vi "Test SigMan Control.vi"() -> ()   [LabVIEW 2020]
uses:
  Controls/SignalManager/SignalManager.xctl
  Classes/SignalManager/SignalManager.lvclass
  Controls/SignalManager/PeriodDisplay.ctl
  Classes/SignalManager/SignalManager.lvclass/SignalManager.ctl
  Classes/SignalManager/Read Error.vi
panel:
  in  "Frame (ms)":dbl
  out "Elapsed time (ms)":u32
  out "Graph":dbl[][](graph)
  out "Error":string
  in  "Read":bool
  in  "Write":bool
  in  "stop":bool
  in  "SigMan":refnum<class "SignalManager.lvclass">(xcontrol)
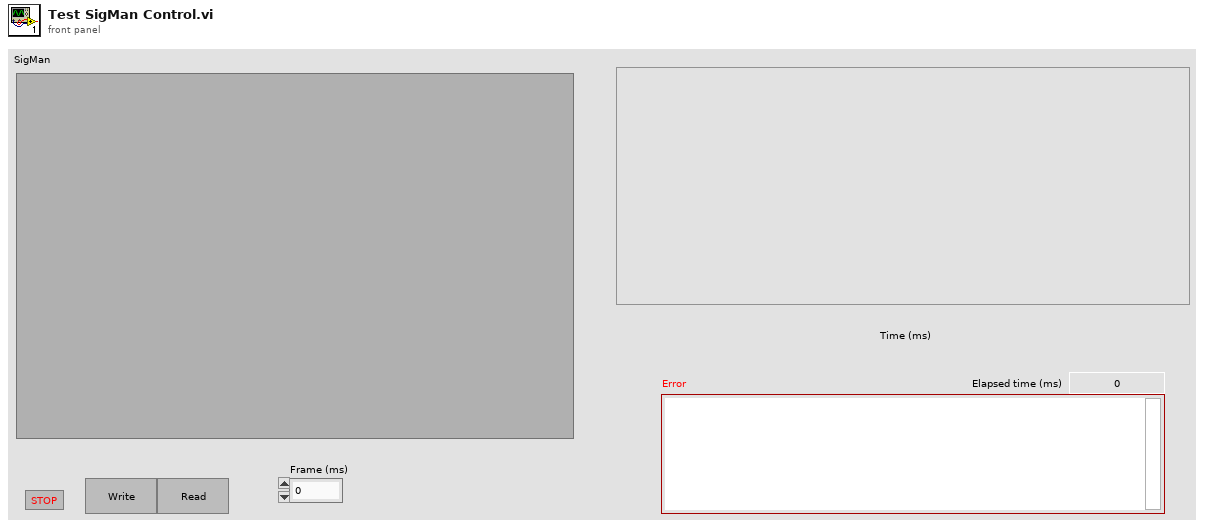
[diagram p1: front panel]
types:
  T1 = typedef "SignalManager.xctl/PeriodDisplay.ctl" = enum16{"Interval", "RepRate", "Both"}
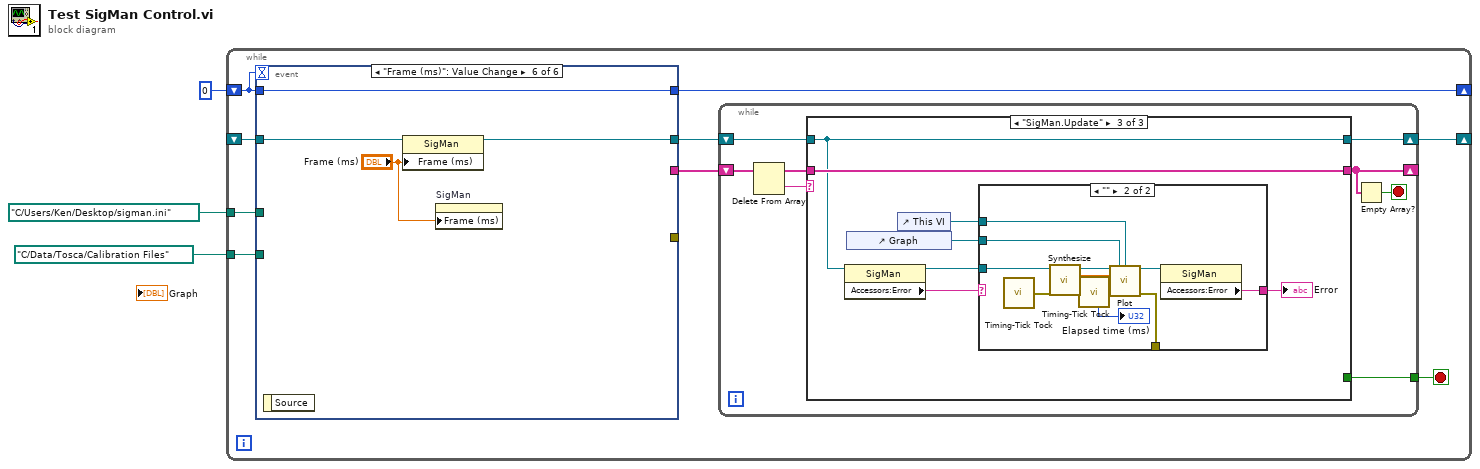
[diagram p0: block diagram]
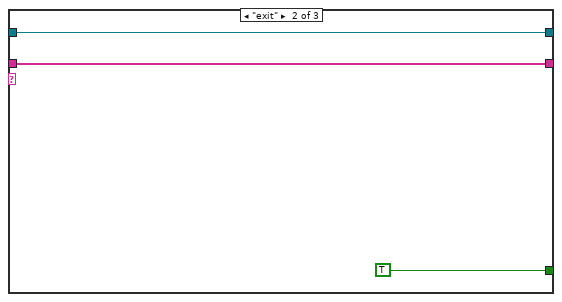
[diagram p3: hidden frame]
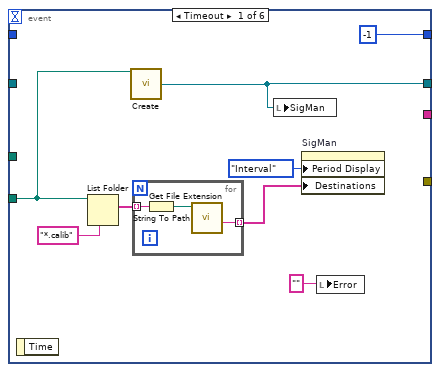
[diagram p5: hidden frame]
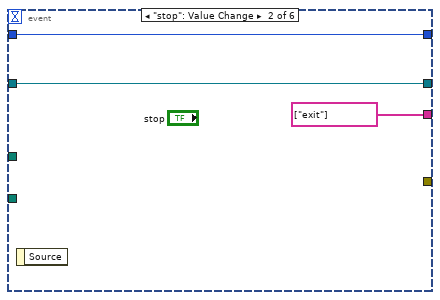
[diagram p6: hidden frame]
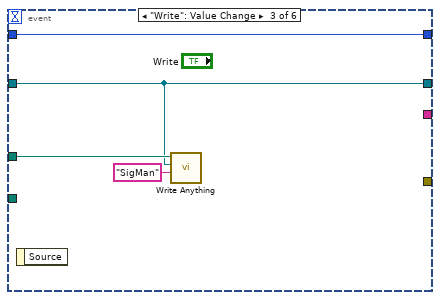
[diagram p7: hidden frame]
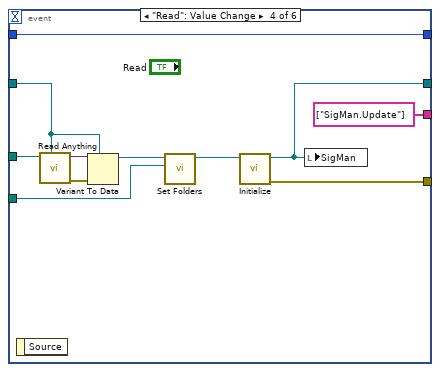
[diagram p8: hidden frame]
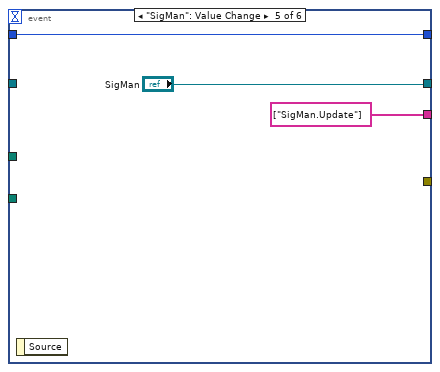
[diagram p9: hidden frame]
diagram:
  n1 = while {
    shift-right: [w11] -> _
    shift-left: 0 -> [w12]
    tunnel: path "C:/Users/Ken/Desktop/sigman.ini" ("Path (dialog)") -> [w10]
    shift-right: [w7] -> _
    shift-left: _ -> [w6]
    tunnel: path "C:/Data/Tosca/Calibration Files" ("Path (dialog)") -> [w4]
    stop <- w5 stop-if-true
    n2 = event shown="[5] \"Frame (ms)\": Value Change" {
      selector: _ -> [_ _ _ _ _ _]
      dyn-events: _ -> [_ _ _ _ _ _]
      timeout: w12 -> [_ _ _ _ _ _]
      tunnel: w12 -> [_ w59 w63 w74 w77 w81]
      tunnel: [-1 w59 w63 w74 w77 w81] -> w11
      tunnel: w10 -> [_ _ w62 w73 _ _]
      tunnel: [w51 w57 w61 w68 "SigMan" w79] -> w8
      tunnel: [_ string[] ["exit"] _ string[] ["SigMan.Update"] string[] ["SigMan.Update"] _] -> w9
      tunnel: w6 -> [_ w57 w61 w70 _ w80]
      tunnel: w4 -> [w50 _ _ w64 _ _]
      tunnel: [_ _ _ w67 _ _] -> _
      event Timeout {
        n3 = event-data() -> ()  [unwired: 1 in, 1 out]
        n4 = List Folder(path=w50, pattern="*.calib") -> (filenames=w48:string[])  [unwired: 2 in, 3 out]
        n5 = call "Create.vi"("Cal Folder"=w50) -> ("SigMan"=w51:refnum<class "SignalManager.lvclass">)  [unwired: 14 in]
        n6 = for {
          tunnel: w48 -> [w55] mode=indexing
          tunnel: [w56] -> w47 mode=indexing
          n7 = String To Path(string=w55) -> (path=w54:path)
          n8 = call <vilib>:"Get File Extension.vi"("file"=w54) -> ("filename without extension"=w56:string)  [unwired: 6 in, 4 out]
        }
        n9 = local write "SigMan"(w51) -> ()
        n10 = property on="SigMan" class="SignalManager (strict)"("Period Display"=PeriodDisplay."Interval", "Destinations"=w47) -> ()  [unwired: 2 in, 2 out]
        n11 = local write "Error"("" ("Error")) -> ()
      }
      event "stop": Value Change {
        n12 = event-data() -> ()  [unwired: 1 in, 1 out]
      }
      event "Write": Value Change {
        n13 = event-data() -> ()  [unwired: 1 in, 1 out]
        n14 = call "Write Anything.vi"("Section Name (Name of \"Anything\")"="SigMan" ("Section Name (Name of \"Anything\")"), "Anything"=w61, "Path (dialog)"=w62) -> ()  [unwired: 7 in, 2 out]
      }
      event "Read": Value Change {
        n15 = event-data() -> ()  [unwired: 1 in, 1 out]
        n16 = call "Read Anything.vi"("Type of Anything"=w70, "Path (dialog)"=w73) -> ("Error Out"=w72:errorcluster, "Anything"=w71:variant)  [unwired: 7 in, 1 out]
        n17 = Variant To Data(error in=w72, type=w70, Variant=w71) -> (data=w66:refnum<class "SignalManager.lvclass">)  [unwired: 1 out]
        n18 = call "Set Folders.vi"("Calibration folder"=w64, "SigMan in"=w66) -> ("SigMan out"=w65:refnum<class "SignalManager.lvclass">)  [unwired: 8 in, 1 out]
        n19 = call "Initialize.vi"("SigMan in"=w65) -> ("error out"=w67:errorcluster, "SigMan out"=w68:refnum<class "SignalManager.lvclass">)  [unwired: 9 in]
        n20 = local write "SigMan"(w68) -> ()
      }
      event "SigMan": Value Change {
        n21 = event-data() -> ()  [unwired: 1 in, 1 out]
      }
      event "Frame (ms)": Value Change {
        n22 = event-data() -> ()  [unwired: 1 in, 1 out]
        n23 = property class="SigMan"(reference=w80, "Frame (ms)"="Frame (ms)") -> (reference out=w79:refnum<class "SignalManager.lvclass">)  [unwired: 1 in, 1 out]
        n24 = property on="SigMan" class="SignalManager (strict)"("Frame (ms)"="Frame (ms)") -> ()  [unwired: 2 in, 2 out]
      }
    }
    n25 = while {
      shift-right: [w17] -> _
      shift-left: w9 -> [w20]
      shift-right: [w14] -> w7
      shift-left: w8 -> [w15]
      tunnel: [w13] -> w5
      stop <- w16 stop-if-true
      n26 = Delete From Array(array=w20) -> (deleted portion=w18:string, array with subset deleted=w19:string[])  [unwired: 2 in]
      n27 = case shown="\"SigMan.Update\"" w18 {
        tunnel: w19 -> [w22 w25 w32]
        tunnel: [w22 w25 w32] -> w17
        tunnel: w15 -> [w21 w24 w31]
        tunnel: [w21 w24 w31] -> w14
        tunnel: [_ TRUE _] -> w13
        frame "", Default {
        }
        frame "exit" {
        }
        frame "SigMan.Update" {
          n28 = property class="SigMan"(reference=w31) -> (reference out=w29:refnum<class "SignalManager.lvclass">, "Accessors:Error"=w30:string)  [unwired: 1 in, 1 out]
          n29 = control-ref of="Graph"() -> (w28:refnum<vi>)
          n30 = control-ref of="This VI"() -> (w27:refnum<vi>)
          n31 = case shown="\"\"" w30 {
            selector: w30 -> [w33 _]
            tunnel: w29 -> [_ w45]
            tunnel: w28 -> [_ w42]
            tunnel: w27 -> [_ w41]
            tunnel: [w33 w38] -> w26
            tunnel: [_ w37] -> _
            frame "error", Default {
            }
            frame "" {
              n32 = call "Timing-Tick Tock.vi"() -> ("error out"=w36:errorcluster)  [unwired: 6 in, 1 out]
              n33 = call "Synthesize.vi"("error in (no error)"=w36, "SigMan in"=w45) -> ("error out"=w40:errorcluster, "Array"=w43:dbl[][], "SigMan out"=w44:refnum<class "SignalManager.lvclass">)  [unwired: 7 in]
              n34 = call "Timing-Tick Tock.vi"("error in (no error)"=w40) -> ("Elapsed time (ms)"=→"Elapsed time (ms)":u32, "error out"=w35:errorcluster)  [unwired: 5 in]
              n35 = call "Plot.vi"("SigMan in"=w44, "Graph"=w42, "VI"=w41, "Array"=w43, "error in (no error)"=w35) -> ("SigMan out"=w39:refnum<class "SignalManager.lvclass">, "error out"=w37:errorcluster)  [unwired: 9 in]
              n36 = property class="SigMan"(reference=w39) -> ("Accessors:Error"=w38:string)  [unwired: 1 in, 2 out]
            }
          }
          "Error" <- w26
        }
      }
      n37 = Empty Array?(array=w17) -> (empty?=w16:bool)
    }
  }
